vi "3458A Get Capabilities.vi"(8 "error in":errorcluster, 9 "Ts [s]":dbl, 10 "aperture [s]":dbl, 11 "digitizer session in":T2 {"channels"."Range [Vpk]" min=0.0}) -> (0 "error out":errorcluster, 2 "capabilities":T1, 3 "digitizer session out":T2 {"channels"."Range [Vpk]" min=0.0})   [LabVIEW 2018, in "3458A Virtual Digitizer.lvlib"]
doc: "This will return capabilities of selected HW. To make it work the session must contain valid setup of the channels and must also contain output of the 'Initialize Virtual Channels' VI, i.e. it may be calle either within opened session or even after the session was closed, because the data produced by 'Initialize Virtual Channels' stay in the session."
uses:
  3458A Virtual Digitizer.lvlib
  3458A Digitizer Session.ctl
  3458A Virtual Channel Config.ctl
  Counter/Counter Session.ctl
  Counter/Counter Type.ctl
  AWG/AWG Session.ctl
  AWG/AWG Type.ctl
  3458A Sync Mode.ctl
  3458A Idn Mode.ctl
  3458A Digitizing Low Levels/Configure/Sampling Mode.ctl
  3458A Digitizing Process Options.ctl
  3458A Data Packet.ctl
  3458A Aux Record Data.ctl
  3458A Digitizing Low Levels/Configure/Level Setup.ctl
  3458A Digitizing Low Levels/Configure/First Sample Trigger.ctl
  3458A Aperture Selection Mode.ctl
  3458A Capabilities.ctl
  <vilib>/Utility/error.llb/Error Cluster From Error Code.vi
  <vilib>/ErrorRing/Error Ring.xnode
  3458A Digitizing Low Levels/3458A Digitizing Low Levels.lvlib
  Counter/Counter.lvlib
  AWG/AWG.lvlib
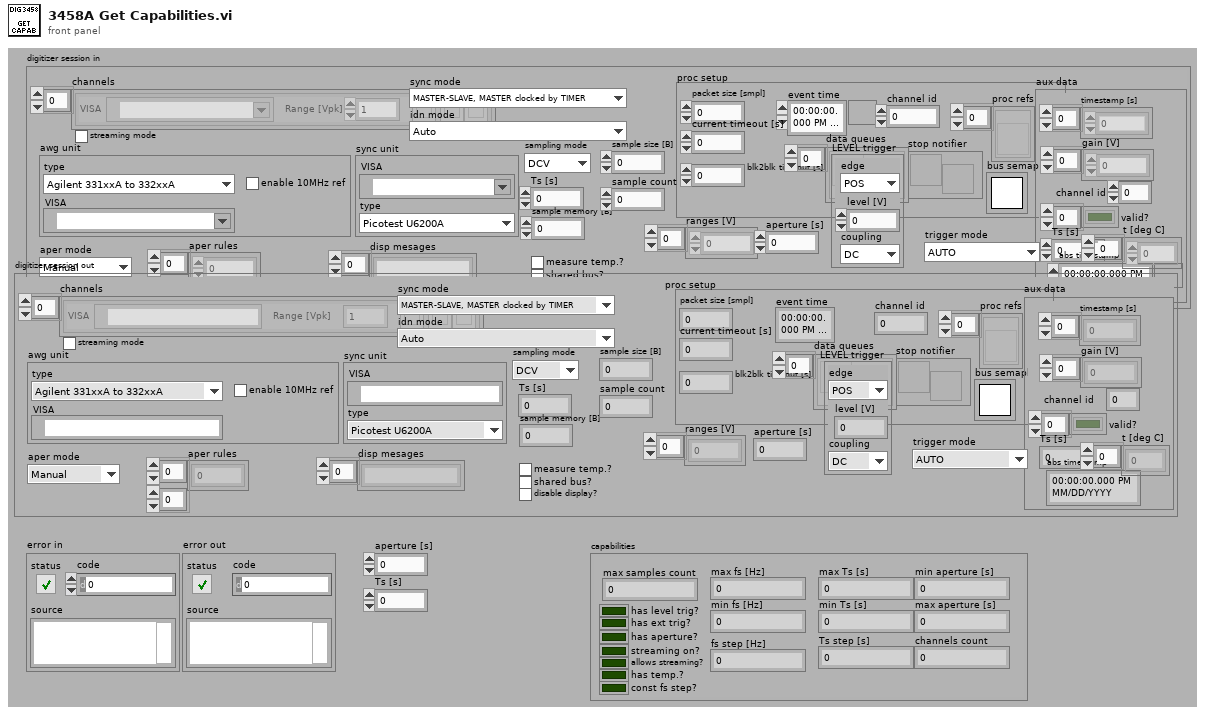
[diagram p1: front panel]
types:
  T1 = typedef "3458A Virtual Digitizer.lvlib/3458A Capabilities.ctl" = cluster{"max samples count":i64, "max fs [Hz]":ext, "min fs [Hz]":ext, "Ts step [s]":ext, "max Ts [s]":ext, "min Ts [s]":ext, "allows streaming?":bool, "streaming on?":bool, "has level trig?":bool, "has ext trig?":bool, "min aperture [s]":dbl, "max aperture [s]":dbl, "has aperture?":bool, "channels count":i32, "has temp.?":bool, "fs step [Hz]":ext, "const fs step?":bool}
  T2 = typedef "3458A Virtual Digitizer.lvlib/3458A Digitizer Session.ctl" = cluster{"channels":T3[], "sync unit":T4, "awg unit":T6, "sync mode":T8, "streaming mode":bool, "idn mode":T9, "sampling mode":T10, "Ts [s]":dbl, "sample memory [B]":i32, "proc setup":T11, "sample size [B]":i32, "sample count":i32, "aux data":T13, "ranges [V]":dbl[], "aperture [s]":dbl, "LEVEL trigger":T14, "trigger mode":T15, "measure temp.?":bool, "disp mesages":string[], "shared bus?":bool, "disable display?":bool, "aper mode":T16, "aper rules":dbl[][]}
  T3 = typedef "3458A Virtual Digitizer.lvlib/3458A Virtual Channel Config.ctl" = cluster{"VISA":refnum<visa-resource-name>, "Range [Vpk]":dbl, "btn clr":bool, "btn up":bool, "btn down":bool}
  T4 = typedef "Counter.lvlib/Counter Session.ctl" = cluster{"VISA":refnum<visa-resource-name>, "type":T5}
  T5 = typedef "Counter.lvlib/Counter Type.ctl" = enum16{"Picotest U6200A", "dummy"}
  T6 = typedef "AWG.lvlib/AWG Session.ctl" = cluster{"type":T7, "VISA":refnum<visa-resource-name>, "enable 10MHz ref":bool}
  T7 = typedef "AWG.lvlib/AWG Type.ctl" = enum16{"Agilent 331xxA to 332xxA", "Agilent 335xxA to 336xxA", "Tektronix AFG3101C", "dummy"}
  T8 = typedef "3458A Virtual Digitizer.lvlib/3458A Sync Mode.ctl" = enum16{"MASTER-SLAVE, MASTER clocked by TIMER", "MASTER-SLAVE, MASTER clocked by AWG", "ALL clocked by AWG", "MASTER-SLAVE, ALL clocked by TIMER", "ALL clocked by AWG with DFLL"}
  T9 = typedef "3458A Virtual Digitizer.lvlib/3458A Idn Mode.ctl" = enum16{"Auto", "Sequential (chn A, chn B, ...)", "From calibration string"}
  T10 = typedef "3458A Virtual Digitizer.lvlib/3458A Digitizing Low Levels.lvlib/Sampling Mode.ctl" = enum16{"DCV", "DSDC", "DSAC"}
  T11 = typedef "3458A Virtual Digitizer.lvlib/3458A Digitizing Process Options.ctl" = cluster{"channel id":i32, "packet size [smpl]":i32, "current timeout [s]":dbl, "blk2blk timeout [s]":dbl, "event time":timestamp, "stop notifier":refnum<notifier>, "data queues":refnum<queue>[], "proc refs":refnum<vi>[], "bus semaphore":T12}
  T12 = typedef "Semaphore RefNum" = refnum<k1>
  T13 = typedef "3458A Virtual Digitizer.lvlib/3458A Aux Record Data.ctl" = cluster{"channel id":i32, "valid?":bool[], "gain [V]":dbl[], "timestamp [s]":dbl[], "Ts [s]":dbl, "abs timestamp":timestamp, "t [deg C]":dbl[]}
  T14 = typedef "3458A Virtual Digitizer.lvlib/3458A Digitizing Low Levels.lvlib/Level Setup.ctl" = cluster{"edge":enum16{"POS", "NEG"}, "level [V]":dbl, "coupling":enum16{"DC", "AC"}}
  T15 = typedef "3458A Virtual Digitizer.lvlib/3458A Digitizing Low Levels.lvlib/First Sample Trigger.ctl" = enum16{"AUTO", "EXT", "SYN", "SGL", "HOLD", "LEVEL"}
  T16 = typedef "3458A Virtual Digitizer.lvlib/3458A Aperture Selection Mode.ctl" = enum16{"Manual", "Maximum", "Table"}
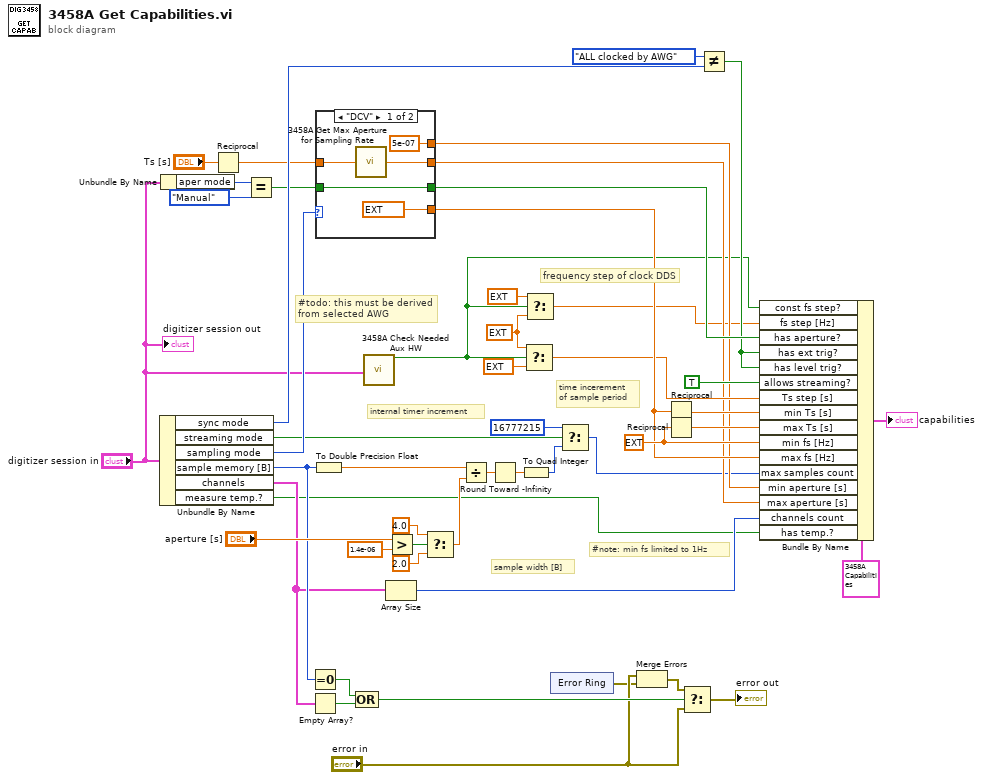
[diagram p0: block diagram]
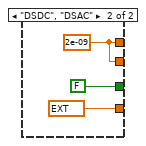
[diagram p2: hidden frame]
diagram:
  w38 = ext 1.0 ("min fs [Hz]")
  w8 = ext nan ("t")
  # "frequency step of clock DDS"
  # "#note: min fs limited to 1Hz"
  # "time incerement\nof sample period"
  # "internal timer increment"
  # "#todo: this must be derived\nfrom selected AWG"
  # "sample width [B]"
  n1 = Unbundle By Name("digitizer session in") -> ("sync mode"=w13:T8, "streaming mode"=w17:bool, "sampling mode"=w41:T10, "sample memory [B]"=w29:i32, "channels"=w20:T3[], "measure temp.?"=w18:bool)
  n2 = Unbundle By Name("digitizer session in") -> ("aper mode"=w3:T16)
  n3 = Reciprocal(x="Ts [s]") -> (1/x=w4:dbl)
  n4 = Equal?(x=w3, y=3458A_Aperture_Selection_Mode."Manual") -> (x = y?=w1:bool)
  n5 = Equal To 0?(x=w29) -> (x = 0?=w30:bool)
  n6 = Empty Array?(array=w20) -> (empty?=w31:bool)
  n7 = To Double Precision Float(number=w29) -> (double precision float=w50:dbl)
  n8 = case shown="\"DCV\"" w41 {
    tunnel: [ext 100000.0 ext 50000.0] -> w35
    tunnel: [w51 FALSE ("allows streaming?")] -> w23
    tunnel: [5e-07 ("min aperture [s]") w56] -> w22
    tunnel: [w53 w56] -> w21
    tunnel: w4 -> [w52 _]
    tunnel: w1 -> [w51 _]
    frame "DCV" {
      n9 = call "3458A Get Max Aperture for Sampling Rate.vi"("fs [Hz]"=w52) -> ("ta_max [s]"=w53:dbl)
    }
    frame "DSDC", "DSAC" {
      w56 = 2e-09 ("min aperture [s]")
    }
  }
  n10 = Compound Arithmetic op=OR(w30, w31) -> (w28:bool)
  n11 = call "3458A Check Needed Aux HW.vi"("digitizer session"="digitizer session in") -> ("uses AWG clocking?"=w7:bool)  [unwired: 13 in, 5 out]
  n12 = Array Size(array=w20) -> (size(s)=w19:i32)
  n13 = Greater?(x="aperture [s]", y=1.4e-06) -> (0:w48:bool)
  n14 = Select(t=4.0, s=w48, f=2.0) -> (s? t:f=w44:dbl)
  n15 = Divide(x=w50, y=w44) -> (x/y=w43:dbl)
  n16 = Round Toward -Infinity(1:w43) -> (0:w42:dbl)
  n17 = To Quad Integer(1:w42) -> (0:w16:i64)
  n18 = Select(t=w8, s=w7, f=ext 1e-7) -> (s? t:f=w34:ext)
  n19 = Select(t=ext 0.0001, s=w7, f=w8) -> (s? t:f=w10:ext)
  n20 = xnode "Error Ring"() -> ("error out"=w24:errorcluster)
  n21 = Select(t=i64 16777215, s=w17, f=w16) -> (s? t:f=w15:i64)
  n22 = Merge Errors("error in", w24) -> (w27:errorcluster)
  n23 = Reciprocal(x=w35) -> (1/x=w36:ext)
  n24 = Reciprocal(x=w38) -> (1/x=w37:ext)
  n25 = Select(t=w27, s=w28, f="error in") -> (s? t:f=→"error out":errorcluster)
  n26 = Not Equal?(x=3458A_Sync_Mode."ALL clocked by AWG", y=w13) -> (x != y?=w11:bool)
  n27 = Bundle By Name(cluster=T1 {"max samples count"=0, "max fs [Hz]"=0.0, "min fs [Hz]"=0.0, "Ts step [s]"=0.0, "max Ts [s]"=0.0, "min Ts [s]"=0.0, "allows streaming?"=FALSE, "streaming on?"=FALSE, "has level trig?"=FALSE, "has ext trig?"=FALSE, "min aperture [s]"=0.0, "max aperture [s]"=0.0, "has aperture?"=FALSE, "channels count"=0, "has temp.?"=FALSE, "fs step [Hz]"=0.0, "const fs step?"=FALSE} ("capabilities"), "const fs step?"=w7, "fs step [Hz]"=w10, "has aperture?"=w23, "has ext trig?"=w11, "has level trig?"=w11, "allows streaming?"=TRUE, "Ts step [s]"=w34, "min Ts [s]"=w36, "max Ts [s]"=w37, "min fs [Hz]"=w38, "max fs [Hz]"=w35, "max samples count"=w15, "min aperture [s]"=w22, "max aperture [s]"=w21, "channels count"=w19, "has temp.?"=w18) -> (→"capabilities":T1)
  "digitizer session out" <- "digitizer session in"
